vi "消解压力计算.vi"(11 "当前消解温度":dbl) -> (3 "消解压力":dbl)   [LabVIEW 2016, in "斯坦道CODCr.lvlib"]
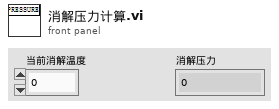
[diagram p1: front panel]
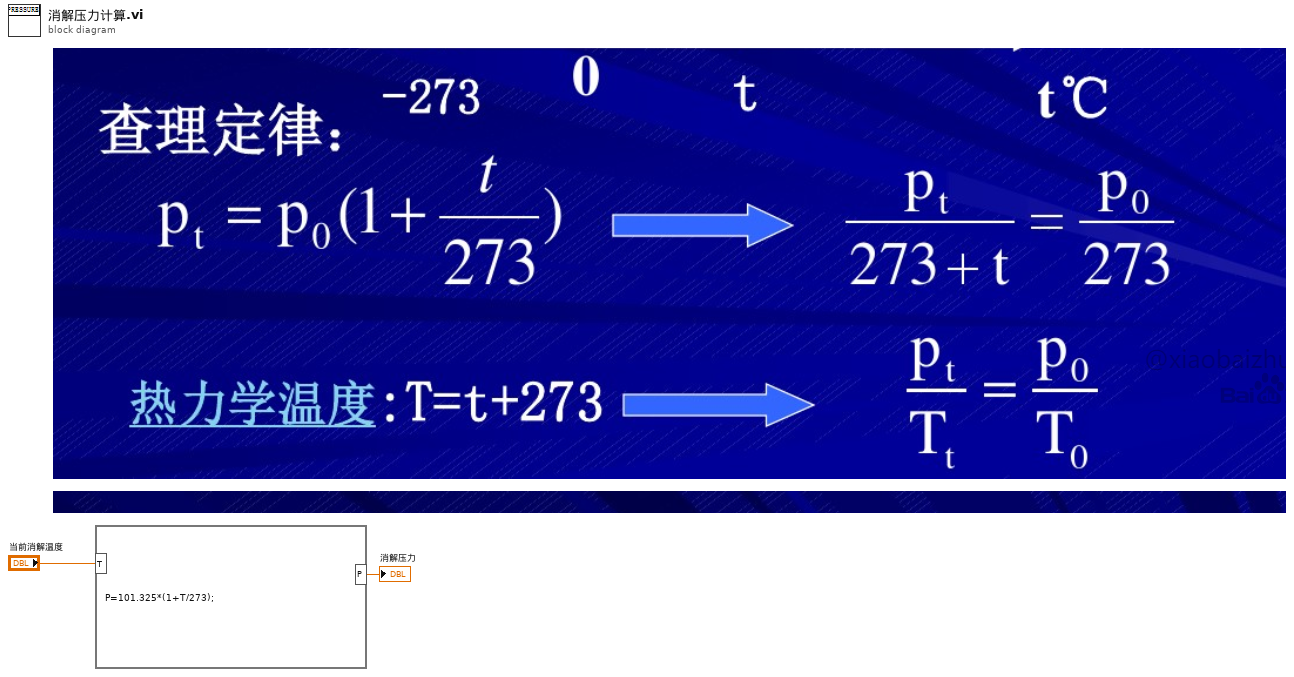
[diagram p0: block diagram]
diagram:
  n1 = formula code="P=101.325*(1+T/273);"("T"="当前消解温度") -> ("P"=→"消解压力":dbl)
